vi "TestExecuteTimedAvgSubscription_PublishOK.vi"(8 "error in (no error)":errorcluster, 11 "TestCase in":refnum<class "TestSubscriptionPolicy.lvclass">) -> (0 "error out":errorcluster, 3 "TestCase out":refnum<class "TestSubscriptionPolicy.lvclass">)   [LabVIEW 2017, in "TestSubscriptionPolicy.lvclass"]
uses:
  TestSubscriptionPolicy.lvclass
  TimedAverageSubscription/TimedAverageSubscription.lvclass/TimedAverageSubscription.ctl
  Transport/QueueTransport/QueueTransport.lvclass/QueueTransport.ctl
  IMediator/ISubscriptionPolicy/ISubscriptionPolicy.lvclass/ISubscriptionPolicy.ctl
  Transport/QueueTransport/QueueTransport.lvclass
  C:/Git/mva-framework/Framework/IMediator/ITransport/ITransport.lvclass
  TimedAverageSubscription/TimedAverageSubscription.lvclass
  C:/Git/mva-framework/Framework/IMediator/ISubscriptionPolicy/ISubscriptionPolicy.lvclass
  <vilib>/Utility/error.llb/Error Cluster From Error Code.vi
  <vilib>/Composed Systems/Timed Average Buffer/New Timed Average Buffer.vi
  IMediator/ISubscriptionPolicy/ISubscriptionPolicy.lvclass
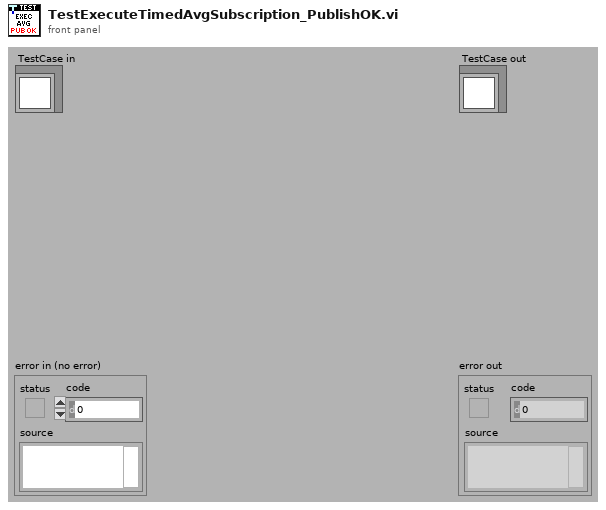
[diagram p1: front panel]
types:
  T1 = typedef "IMediator.lvlib/ISubscriptionPolicy.lvclass/ISubscriptionPolicy Reference.ctl" = refnum<data-value>
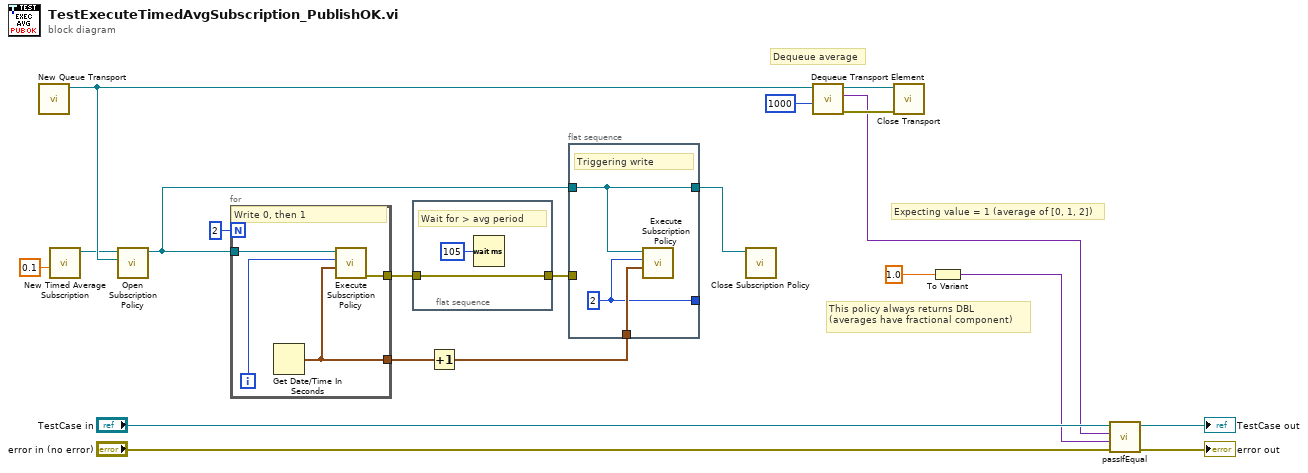
[diagram p0: block diagram]
diagram:
  # "This policy always returns DBL\n(averages have fractional component)"
  # "Dequeue average"
  # "Expecting value = 1 (average of [0, 1, 2])"
  n1 = call "New Queue Transport.vi"() -> ("QueueTransport"=w16:refnum<class "QueueTransport.lvclass">)  [unwired: 10 in, 1 out]
  n2 = call "New Timed Average Subscription.vi"("Average Period [s]"=0.1) -> ("TimedAverageSubscription Out"=w12:refnum<class "TimedAverageSubscription.lvclass">)  [unwired: 10 in]
  n3 = call "Open Subscription Policy.vi"("Transport"=w16, "SubscriptionPolicy"=w12) -> ("Subscription Policy"=w11:T1)  [unwired: 8 in, 1 out]
  n4 = for {
    N: 2 -> [_]
    tunnel: w11 -> [w24]
    tunnel: [w23] -> w10
    tunnel: [w22] -> w4
    i -> [w21]
    # "Write 0, then 1"
    n5 = Get Date/Time In Seconds() -> (seconds since 1Jan1904=w23:timestamp)
    n6 = call "Execute Subscription Policy.vi"("Publish Time"=w23, "New Topic Value"=w21, "Subscription Policy"=w24) -> ("error out (Unsubscribe?)"=w22:errorcluster)  [unwired: 8 in]
  }
  n7 = flat-sequence {
    tunnel: w4 -> [w26]
    tunnel: [w26] -> w3
    frame #0 {
      # "Wait for > avg period"
      n8 = Wait (ms)(milliseconds to wait=u32 105) -> ()  [unwired: 1 out]
    }
  }
  n9 = Increment(x=w10) -> (x+1=w9:timestamp)
  n10 = flat-sequence {
    tunnel: w11 -> [w27]
    tunnel: w9 -> [w29]
    tunnel: [w28] -> _
    tunnel: w3 -> [_]
    tunnel: [w27] -> w2
    frame #0 {
      w28 = 2
      # "Triggering write"
      n11 = call "Execute Subscription Policy.vi"("Publish Time"=w29, "New Topic Value"=w28, "Subscription Policy"=w27) -> ()  [unwired: 8 in, 1 out]
    }
  }
  n12 = call "Close Subscription Policy.vi"("Subscription Policy Reference"=w2) -> ()  [unwired: 10 in, 1 out]
  n13 = call "Dequeue Transport Element.vi"("Timeout In ms (-1)"=1000, "QueueTransport in"=w16) -> ("error out"=w13:errorcluster, "Data"=w1:variant, "QueueTransport out"=w14:refnum<class "QueueTransport.lvclass">)  [unwired: 6 in, 1 out]
  n14 = call-dynamic "Close Transport.vi"("error in (no error)"=w13, "QueueTransport in"=w14) -> ()  [unwired: 9 in, 1 out]
  n15 = To Variant(anything=1.0) -> (Variant=w5:variant)
  n16 = call-dynamic "passIfEqual.vi"("error in (no error)"="error in (no error)", "y"=w5, "x"=w1, "TestCase in"="TestCase in") -> ("error out"=→"error out":errorcluster, "TestCase out"=→"TestCase out":refnum<class "TestSubscriptionPolicy.lvclass">)  [unwired: 6 in]
